vi "APLUS Watt Hours.vi"(8 "error in (no error)":errorcluster, 11 "Modbus instance in":refnum<class "Modbus API.lvclass">) -> (0 "error out":errorcluster, 3 "Modbus instance out":refnum<class "Modbus API.lvclass">, 5 "Watt Hours":dbl)   [LabVIEW 2019]
uses:
  <vilib>/NI/Modbus Library/API/Modbus API.lvclass
  Type Definitions/APLUS Commands.ctl
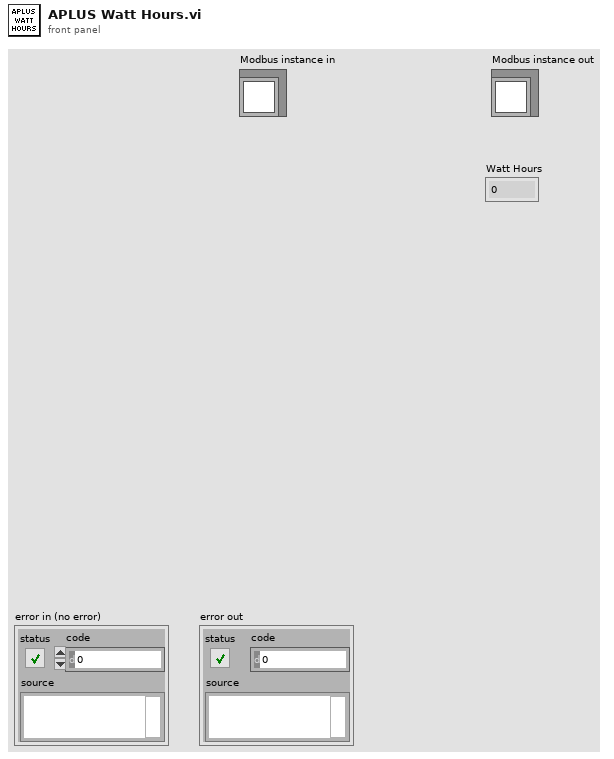
[diagram p1: front panel]
types:
  T1 = typedef "APLUS Commands.ctl" = u16
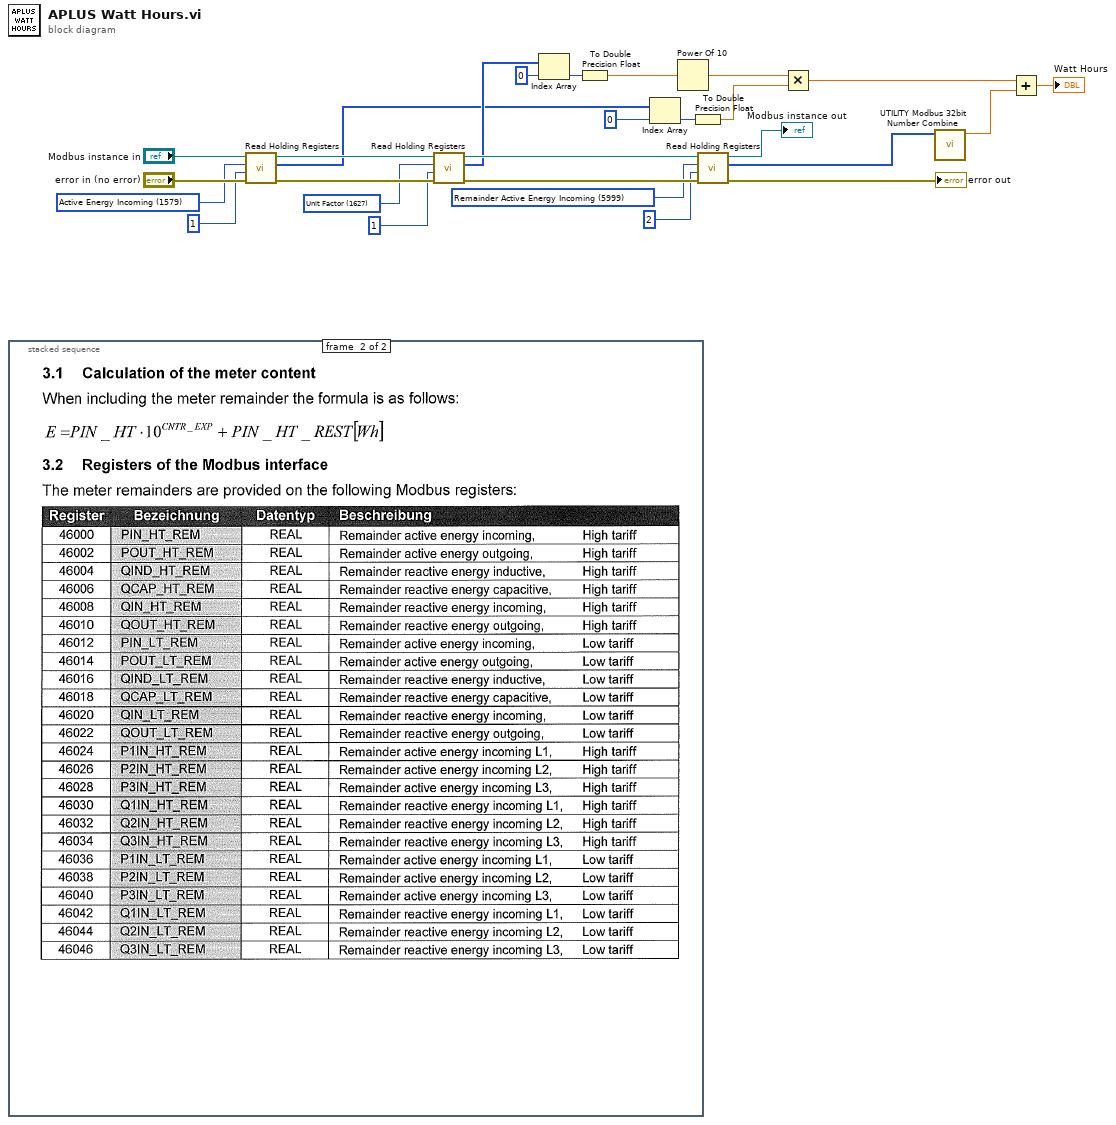
[diagram p0: block diagram]
diagram:
  w1 = T1 5999 items=["Voltage (V)"=1839, "RMS Current (Amps)"=1841, "Frequency (Hz)"=1843, "Power (Watts)"=1845, "Power Factor"=1847, "Apparent Power (VA)"=1849, "Voltage Total Harmonic Distortion (%)"=1851, "Active Energy Incoming"=1579, "Unit Factor"=1627, "Remainder Active Energy Incoming"=5999] ("APLUS Modbus Registers")
  w2 = T1 1627 items=["Voltage (V)"=1839, "RMS Current (Amps)"=1841, "Frequency (Hz)"=1843, "Power (Watts)"=1845, "Power Factor"=1847, "Apparent Power (VA)"=1849, "Voltage Total Harmonic Distortion (%)"=1851, "Active Energy Incoming"=1579, "Unit Factor"=1627, "Remainder Active Energy Incoming"=5999] ("APLUS Modbus Registers")
  w3 = T1 1579 items=["Voltage (V)"=1839, "RMS Current (Amps)"=1841, "Frequency (Hz)"=1843, "Power (Watts)"=1845, "Power Factor"=1847, "Apparent Power (VA)"=1849, "Voltage Total Harmonic Distortion (%)"=1851, "Active Energy Incoming"=1579, "Unit Factor"=1627, "Remainder Active Energy Incoming"=5999] ("APLUS Modbus Registers")
  n1 = stacked-sequence {
    frame #0 {
    }
    frame #1 {
    }
  }
  n2 = call-dynamic "Read Holding Registers.vi"("error in"="error in (no error)", "number of inputs"=u16 1 ("Quantity"), "starting address"=w3, "Modbus instance in"="Modbus instance in") -> ("error out"=w9:errorcluster, "register values"=w13:u16[], "Modbus instance out"=w15:refnum<class "Modbus API.lvclass">)  [unwired: 5 in]
  n3 = call-dynamic "Read Holding Registers.vi"("error in"=w9, "number of inputs"=u16 1 ("Quantity"), "starting address"=w2, "Modbus instance in"=w15) -> ("error out"=w8:errorcluster, "register values"=w16:u16[], "Modbus instance out"=w18:refnum<class "Modbus API.lvclass">)  [unwired: 5 in]
  n4 = Index Array(array=w16, index=0) -> (element=w20:u16)
  n5 = To Double Precision Float(number=w20) -> (double precision float=w22:dbl)
  n6 = Index Array(array=w13, index=0) -> (element=w27:u16)
  n7 = Power Of 10(x=w22) -> (10^x=w21:dbl)
  n8 = To Double Precision Float(number=w27) -> (double precision float=w23:dbl)
  n9 = call-dynamic "Read Holding Registers.vi"("error in"=w8, "number of inputs"=u16 2 ("Quantity"), "starting address"=w1, "Modbus instance in"=w18) -> ("error out"=→"error out":errorcluster, "register values"=w19:u16[], "Modbus instance out"=→"Modbus instance out":refnum<class "Modbus API.lvclass">)  [unwired: 5 in]
  n10 = Multiply(x=w21, y=w23) -> (x*y=w24:dbl)
  n11 = call "UTILITY Modbus 32bit Number Combine.vi"("Holding Registers"=w19) -> ("Data"=w25:sgl)  [unwired: 9 in, 1 out]
  n12 = Add(x=w24, y=w25) -> (x+y=→"Watt Hours":dbl)
